vi "Actor Core.vi"(8 "error in":errorcluster, 11 "Context in":refnum<class "Context.lvclass">) -> (0 "error out":errorcluster, 3 "Actor out":refnum<class "Actor.lvclass">)   [LabVIEW 2021, in "Context.lvlib" / "Context.lvclass"]
doc: "(<B>Filename</B>: Actor Framework.lvlib:Actor.lvclass:Actor Core.vi)\n\nReceives messages to the actor, reacts to them, and initiates any error handling that may shut the actor down.\n\nDescendant classes may override this VI to append parallel tasks for the actor to complete while it handles messages. Overrides use the Call Parent Class Method node."
uses:
  Context.lvclass
  C:/PPLs/Design-Patterns/State Pattern/State Pattern/State Pattern.lvclass
  C:/Program Files/National Instruments/LabVIEW 2021/vi.lib/ActorFramework/Actor/Actor.lvclass
  <vilib>/ActorFramework/Actor/Actor.lvclass
  Context.lvclass/Context.ctl
  State Pattern/State Pattern.lvclass
  A Context State/A Context State.lvclass
  C:/PPLs/Design-Patterns/State Pattern/Context/Context/Context.lvclass
  C:/PPLs/Design-Patterns/State Pattern/xxxx/xxxx/xxxx.lvclass
  C:/PPLs/Design-Patterns/State Pattern/Context/Context State/Context State.lvclass
  C:/PPLs/Design-Patterns/State Pattern/Context/A Context State/A Context State.lvclass
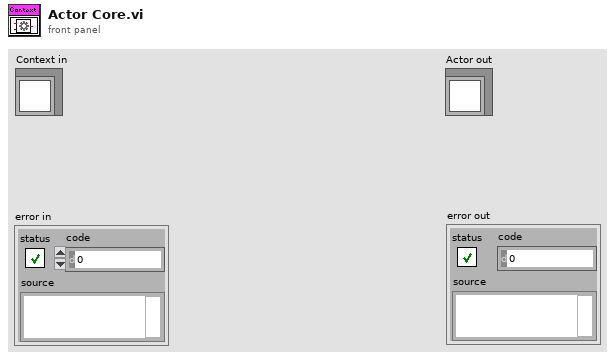
[diagram p1: front panel]
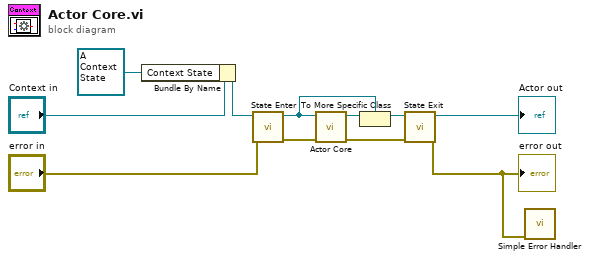
[diagram p0: block diagram]
diagram:
  n1 = Bundle By Name(cluster="Context in", "Context State"=refnum<class "A Context State.lvclass"> refnum ("Context.lvlib:A Context State.lvclass")) -> (w3:refnum<class "Context.lvclass">)
  n2 = call "State Enter.vi"("error in"="error in", "State Pattern in"=w3) -> ("error out"=w9:errorcluster, "State Pattern out"=w4:refnum<class "Context.lvclass">)  [unwired: 8 in]
  n3 = call-parent "Actor Core.vi"("error in"=w9, "Actor in"=w4) -> ("error out"=w6:errorcluster, "Actor out"=w8:refnum<class "Actor.lvclass">)  [unwired: 8 in]
  n4 = To More Specific Class(target class=w4, reference=w8) -> (specific class reference=w5:refnum<class "Context.lvclass">)  [unwired: 1 in, 1 out]
  n5 = call "State Exit.vi"("error in"=w6, "State Pattern in"=w5) -> ("error out"=w1:errorcluster, "State Pattern out"=→"Actor out":refnum<class "Context.lvclass">)  [unwired: 8 in]
  "error out" <- w1
  n6 = call <vilib>:"Simple Error Handler.vi"("error in (no error)"=w1) -> ()  [unwired: 4 in, 5 out]
